vi "peak comb -- interpolate - complex plane - V2.vi"(6 "peaks are known -- parameters":T1={"Def Gamma (kHz)"=0.0, "dV"=0.0, "time in Gamma (sec)"=0.0, "phi-star"=0.0, "all peaks (kHz)"=[564.0, 649.0, 987.0, 1133.0, 1214.0, 1585.0, 1763.0, 1823.0, 1880.0, 1899.0, 2032.0, 2138.0, 2221.0, 2270.0, 2350.0, 2456.0, 2580.0, 2634.0, 2831.0, 2960.0, 2965.0, 3131.0, 3328.0, 3469.0, 3553.0, 0.0, 3615.0, 3734.0, 0.0, 0.0, 0.0, 4236.0, 4300.0, 4331.0], "delta t (sec)"=0.0, "default step (Hz)"=0.0, "Max step (Hz)"=0.0, "all gamma (kHz)"=[564.0, 649.0, 987.0, 1133.0, 1214.0, 1585.0, 1763.0, 1823.0, 1880.0, 1899.0, 2032.0, 2138.0, 2221.0, 2270.0, 2350.0, 2456.0, 2580.0, 2634.0, 2831.0, 2960.0, 2965.0, 3131.0, 3328.0, 3469.0, 3553.0, 0.0, 3615.0, 3734.0, 0.0, 0.0, 0.0, 4236.0, 4300.0, 4331.0], "peaks OK"=FALSE, "gamma OK"=FALSE}, 9 "Gamma (kHz)":dbl=nan, 11 "freq (kHz)":dbl) -> (3 "delta-F (Hz)":dbl=-1.0)   [LabVIEW 2010]
uses:
  next chunk -- parameters.ctl
  Q - not nan -- real.vi
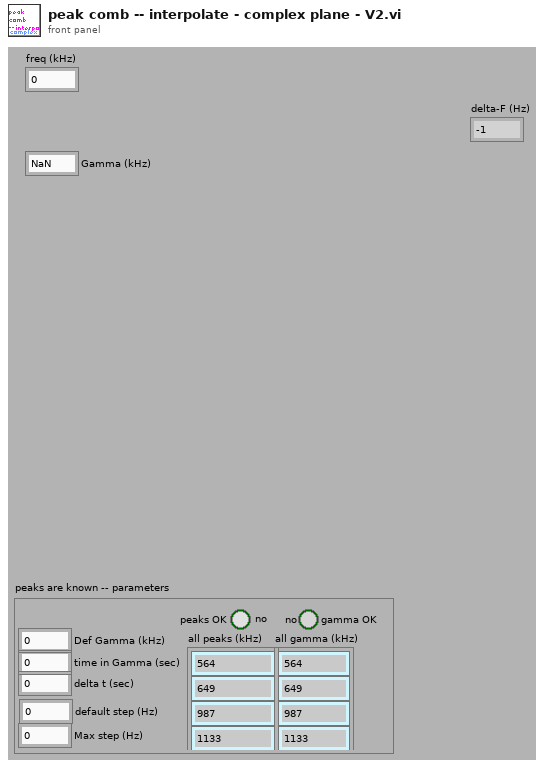
[diagram p1: front panel]
types:
  T1 = typedef "next chunk -- parameters.ctl" = cluster{"Def Gamma (kHz)":dbl, "dV":dbl, "time in Gamma (sec)":dbl, "phi-star":dbl, "all peaks (kHz)":dbl[], "delta t (sec)":dbl, "default step (Hz)":dbl, "Max step (Hz)":dbl, "all gamma (kHz)":dbl[], "peaks OK":bool, "gamma OK":bool}
  T2 = typedef "comparison control.ctl" = enum16{"not a number", "above", "in range", "below"}
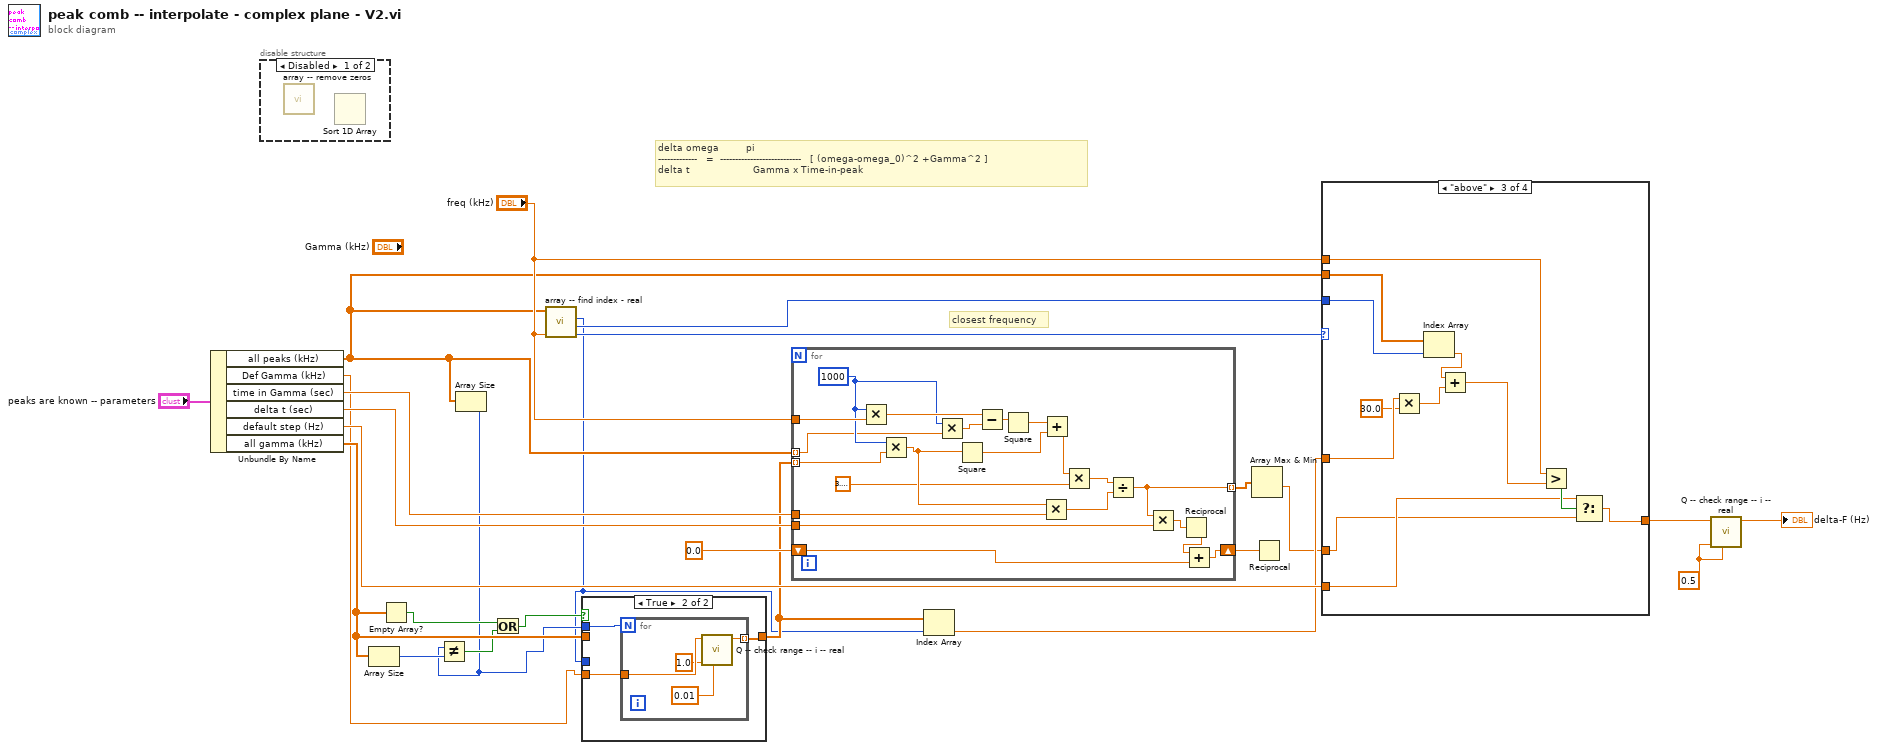
[diagram p0: block diagram]
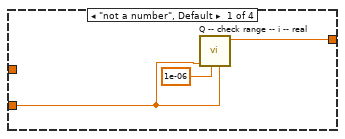
[diagram p4: hidden frame]
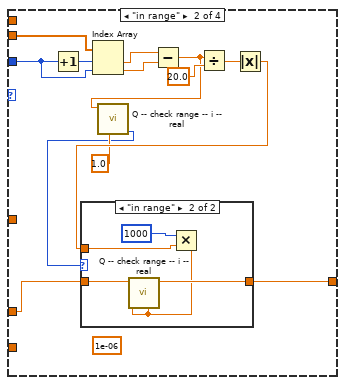
[diagram p5: hidden frame]
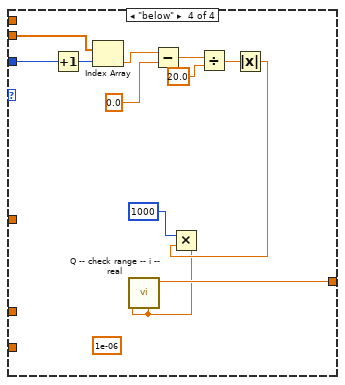
[diagram p7: hidden frame]
diagram:
  w11 = 0.5 ("default")
  # "closest frequency"
  # "delta omega         pi\n-------------   =  ---------------------------   [ (omega-omega_0)^2 +Gamma^2 ] \ndelta t                     Gamma x Time-in-peak"
  n1 = Unbundle By Name("peaks are known -- parameters") -> ("all peaks (kHz)"=w7:dbl[], "Def Gamma (kHz)"=w9:dbl, "time in Gamma (sec)"=w24:dbl, "delta t (sec)"=w23:dbl, "default step (Hz)"=w19:dbl, "all gamma (kHz)"=w18:dbl[])
  n2 = disable-structure shown="Disabled" {
    frame Disabled {
      n3 = call "array -- remove zeros.vi"() -> ()  [unwired: 11 in, 1 out]
      n4 = Sort 1D Array() -> ()  [unwired: 1 in, 1 out]
    }
    frame Enabled {
    }
  }
  n5 = Array Size(array=w18) -> (size(s)=w17:i32)
  n6 = Empty Array?(array=w18) -> (empty?=w16:bool)
  n7 = Array Size(array=w7) -> (size(s)=w10:i32)
  n8 = Not Equal?(x=w10, y=w17) -> (x != y?=w15:bool)
  n9 = Or(x=w16, y=w15) -> (x .or. y?=w14:bool)
  n10 = call "array -- find index - real.vi"("number"="freq (kHz)", "temperatures"=w7) -> ("selector"=w22:T2, "left index"=w21:i32, "closest element index"=w5:i32)  [unwired: 6 in, 1 out]
  n11 = case shown="True" w14 {
    tunnel: w5 -> [_ _]
    tunnel: w18 -> [w26 _]
    tunnel: w10 -> [_ w29]
    tunnel: w9 -> [_ w28]
    tunnel: [w26 w27] -> w6
    frame False {
    }
    frame True {
      n12 = for {
        N: w29 -> [_]
        tunnel: w28 -> [w32]
        tunnel: [w30] -> w27 mode=indexing
        n13 = call "Q -- check range -- i -- real.vi"("lower"=0.01, "default"=1.0, "number"=w32) -> ("number in range"=w30:dbl)  [unwired: 6 in, 2 out]
      }
    }
  }
  n14 = for {
    tunnel: w24 -> [w54]
    tunnel: w23 -> [w53]
    tunnel: "freq (kHz)" -> [w52]
    shift-right: [w36] -> w3
    shift-left: 0.0 ("lower") -> [w35]
    tunnel: w7 -> [w40] mode=indexing
    tunnel: w6 -> [w39] mode=indexing
    tunnel: [w34] -> w2 mode=indexing
    w43 = 1000 ("dimension size")
    n15 = Multiply(x=w43, y=w52) -> (x*y=w45:dbl)
    n16 = Multiply(x=w43, y=w39) -> (x*y=w42:dbl)
    n17 = Multiply(x=w43, y=w40) -> (x*y=w44:dbl)
    n18 = Square(x=w42) -> (x^2=w49:dbl)
    n19 = Subtract(x=w45, y=w44) -> (x-y=w51:dbl)
    n20 = Square(x=w51) -> (x^2=w50:dbl)
    n21 = Multiply(x=w42, y=w54) -> (x*y=w46:dbl)
    n22 = Add(x=w50, y=w49) -> (x+y=w48:dbl)
    n23 = Multiply(x=w48, y=3.141592653589793) -> (x*y=w47:dbl)
    n24 = Divide(x=w47, y=w46) -> (x/y=w34:dbl)
    n25 = Multiply(x=w34, y=w53) -> (x*y=w38:dbl)
    n26 = Reciprocal(x=w38) -> (1/x=w37:dbl)
    n27 = Add(x=w37, y=w35) -> (x+y=w36:dbl)
  }
  n28 = Index Array(array=w6, index=w5) -> (element=w4:dbl)
  n29 = Array Max & Min(array=w2) -> (min value=w1:dbl)  [unwired: 3 out]
  n30 = Reciprocal(x=w3) -> ()  [unwired: 1 out]
  n31 = case shown="\"above\"" w22 {
    tunnel: w21 -> [_ w63 w87 w90]
    tunnel: w7 -> [_ w69 w88 w99]
    tunnel: "freq (kHz)" -> [_ _ w82 _]
    tunnel: [w55 w65 w78 w94] -> w13
    tunnel: w19 -> [w56 _ w79 _]
    tunnel: w4 -> [_ _ w85 _]
    tunnel: w1 -> [_ w61 w77 _]
    frame "not a number", Default {
      n32 = call "Q -- check range -- i -- real.vi"("upper"=w56, "lower"=1e-06, "default"=w56) -> ("number in range"=w55:dbl)  [unwired: 6 in, 2 out]
    }
    frame "in range" {
      (unwired) 1e-06 ("lower")
      n33 = Increment(x=w63) -> (x+1=w70:i32)
      n34 = Index Array(array=w69, index #1=w70, index #2=w63) -> (element #1=w68:dbl, element #2=w62:dbl)
      n35 = Subtract(x=w68, y=w62) -> (x-y=w60:dbl)
      n36 = call "Q -- check range -- i -- real.vi"("lower"=1.0, "number"=w60) -> ("selector"=w58:T2)  [unwired: 7 in, 2 out]
      n37 = Divide(x=w60, y=20.0) -> (x/y=w66:dbl)
      n38 = Absolute Value(x=w66) -> (abs(x)=w64:dbl)
      n39 = case shown="\"in range\"" w58 {
        tunnel: [w71 w76] -> w65
        tunnel: w64 -> [_ w74]
        tunnel: w61 -> [w71 w72]
        frame "not a number", Default {
        }
        frame "in range" {
          n40 = Multiply(x=1000 ("dimension size"), y=w74) -> (x*y=w73:dbl)
          n41 = call "Q -- check range -- i -- real.vi"("upper"=w73, "default"=w73, "number"=w72) -> ("number in range"=w76:dbl)  [unwired: 6 in, 2 out]
        }
      }
    }
    frame "above" {
      n42 = Multiply(x=w85, y=30.0) -> (x*y=w83:dbl)
      n43 = Index Array(array=w88, index=w87) -> (element=w86:dbl)
      n44 = Add(x=w86, y=w83) -> (x+y=w81:dbl)
      n45 = Greater?(x=w82, y=w81) -> (0:w80:bool)
      n46 = Select(t=w79, s=w80, f=w77) -> (s? t:f=w78:dbl)
    }
    frame "below" {
      (unwired) 1e-06 ("lower")
      n47 = Increment(x=w90) -> (x+1=w100:i32)
      n48 = Index Array(array=w99, index=w100) -> (element=w98:dbl)
      n49 = Subtract(x=w98, y=0.0) -> (x-y=w97:dbl)
      n50 = Divide(x=w97, y=20.0) -> (x/y=w95:dbl)
      n51 = Absolute Value(x=w95) -> (abs(x)=w92:dbl)
      n52 = Multiply(x=1000 ("dimension size"), y=w92) -> (x*y=w91:dbl)
      n53 = call "Q -- check range -- i -- real.vi"("upper"=w91, "default"=w91) -> ("number in range"=w94:dbl)  [unwired: 7 in, 2 out]
    }
  }
  n54 = call "Q -- check range -- i -- real.vi"("lower"=w11, "default"=w11, "number"=w13) -> ("number in range"=→"delta-F (Hz)":dbl)  [unwired: 6 in, 2 out]
